vi "close.vi"(8 "error in (no error)":errorcluster, 11 "PsuNiPxi in":refnum<class "PsuNi.lvclass">) -> (0 "error out":errorcluster)   [LabVIEW 2023, in "PsuNi.lvclass"]
doc: "<b>Author:</b> Wolfgang\n<b>Description:</b> This mimics the abilty to close an instrument reference if opened before."
uses:
  PsuNi.lvclass
  PsuNi.lvclass/PsuNi.ctl
  PowerSupply.lvclass
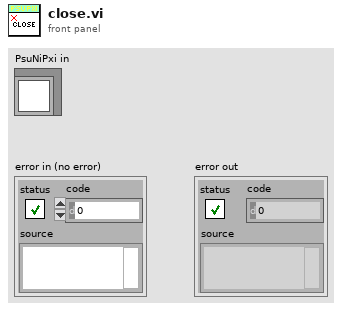
[diagram p1: front panel]
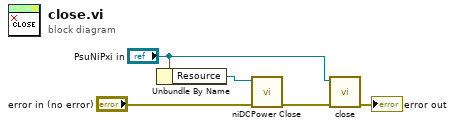
[diagram p0: block diagram]
diagram:
  n1 = Unbundle By Name("PsuNiPxi in") -> ("Resource"=w3:refnum<k15>)
  n2 = call <instrlib>:"niDCPower Close.vi"("error in (no error)"="error in (no error)", "instrument handle"=w3) -> ("error out"=w1:errorcluster)  [unwired: 9 in]
  n3 = call-parent "close.vi"("error in (no error)"=w1, "Instrument in"="PsuNiPxi in") -> ("error out"=→"error out":errorcluster)  [unwired: 9 in]
